vi "Word Insert Object.vi"(0 "report in":refnum<class "NI_report.lvclass">, 5 "file path":path, 7 "bookmark (\"\")":string, 9 "link to file? (F)":bool, 11 "error in (no error)":errorcluster) -> (4 "report out":refnum<class "NI_report.lvclass">, 15 "error out":errorcluster)   [LabVIEW 2020, in "NI_Word.lvclass"]
doc: "Inserts an object associated with a file into the current document."
uses:
  <vilib>/Utility/NIReport.llb/Word/NI_Word.lvclass
  <vilib>/Utility/NIReport.llb/NI_report.lvclass
  C:/Program Files (x86)/National Instruments/LabVIEW 2020/vi.lib/Utility/NIReport.llb/NI_report.lvclass
  <vilib>/Utility/NIReport.llb/Word/NI_Word.lvclass/NI_Word.ctl
  <vilib>/addons/_office/NI_ReportGenerationToolkit.lvlib
  <vilib>/Utility/NIReport.llb/NI_ReportGenerationCore.lvlib
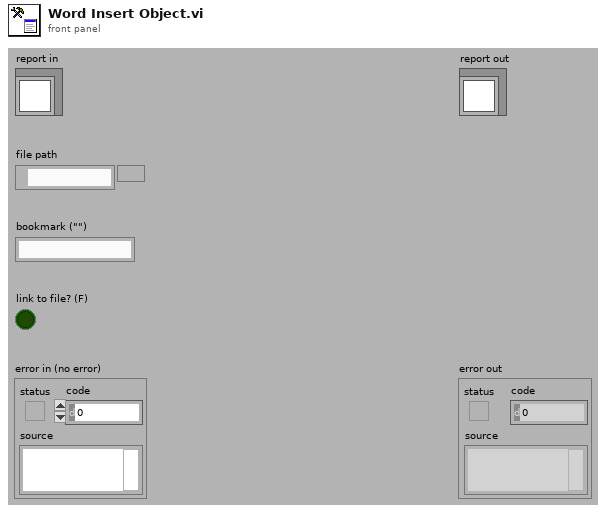
[diagram p1: front panel]
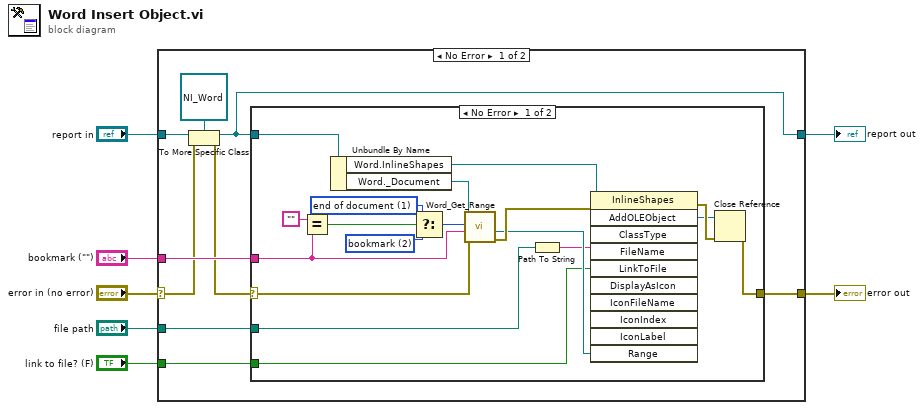
[diagram p0: block diagram]
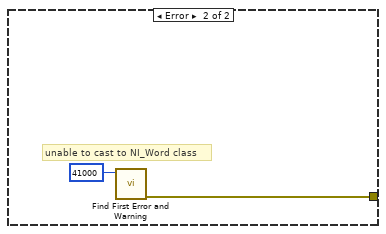
[diagram p2: hidden frame]
diagram:
  n1 = case shown="No Error" "error in (no error)" {
    selector: "error in (no error)" -> [w9 w38]
    tunnel: [w16 w38] -> w6
    tunnel: [w8 w37] -> w4
    tunnel: "report in" -> [w11 w37]
    tunnel: "bookmark (\"\")" -> [w15 _]
    tunnel: "link to file? (F)" -> [w14 _]
    tunnel: "file path" -> [w13 _]
    frame No Error {
      n2 = To More Specific Class(target class=refnum<class "NI_Word.lvclass"> refnum ("report in"), reference=w11, error in=w9) -> (specific class reference=w8:refnum<class "NI_Word.lvclass">, error out=w10:errorcluster)
      n3 = case shown="No Error" w10 {
        selector: w10 -> [w17 _]
        tunnel: [w24 w35] -> w16
        tunnel: w15 -> [w22 _]
        tunnel: w14 -> [w20 _]
        tunnel: w13 -> [w19 _]
        tunnel: w8 -> [w18 _]
        frame No Error {
          w31 = u16 2 items=["begining of document", "end of document", "bookmark", "custom"] ("Insertion point")
          w32 = u16 1 items=["begining of document", "end of document", "bookmark", "custom"] ("Insertion point")
          n4 = Equal?(x="", y=w22) -> (x = y?=w33:bool)
          n5 = Unbundle By Name(w18) -> ("Word.InlineShapes"=w23:refnum<k7>, "Word._Document"=w29:refnum<k7>)
          n6 = Select(t=w32, s=w33, f=w31) -> (s? t:f=w34:u16)
          n7 = call <vilib>:"Word_Get_Range.vi"("error in"=w17, "bookmark name"=w22, "insertion point"=w34, "document in"=w29) -> ("error out (no error)"=w30:errorcluster, "range"=w26:refnum<k7>)  [unwired: 2 in, 4 out]
          n8 = Path To String(path=w19) -> (string=w25:string)
          n9 = invoke class="InlineShapes" method="AddOLEObject"(reference=w23, error in=w30, "FileName"=w25, "LinkToFile"=w20, "Range"=w26) -> (error out=w28:errorcluster, "AddOLEObject"=w27:refnum<k7>)  [unwired: 6 in, 9 out]
          n10 = Close Reference(reference=w27, error in (no error)=w28) -> (error out=w24:errorcluster)
        }
        frame Error {
          # "unable to cast to NI_Word class"
          n11 = call <vilib>:"Find First Error and Warning.vi"("error code"=41000) -> ("error out"=w35:errorcluster)  [unwired: 2 in, 4 out]
        }
      }
    }
    frame Error {
    }
  }
  "error out" <- w6
  "report out" <- w4
